vi "set MIC.maxpower.vi"() -> ()   [LabVIEW 2012]
uses:
  GFG/GFGnumericGet.vi
  GFG/GFG library.lvlib
panel:
  in  "OK Button":bool
  # "set half-wave plate to MAXIMUM power\nusing the control cube"
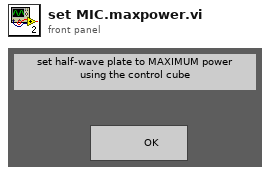
[diagram p1: front panel]
types:
  T1 = enum32{"Invalid", "Standard", "Closed", "Hidden", "Minimized", "Maximized"}
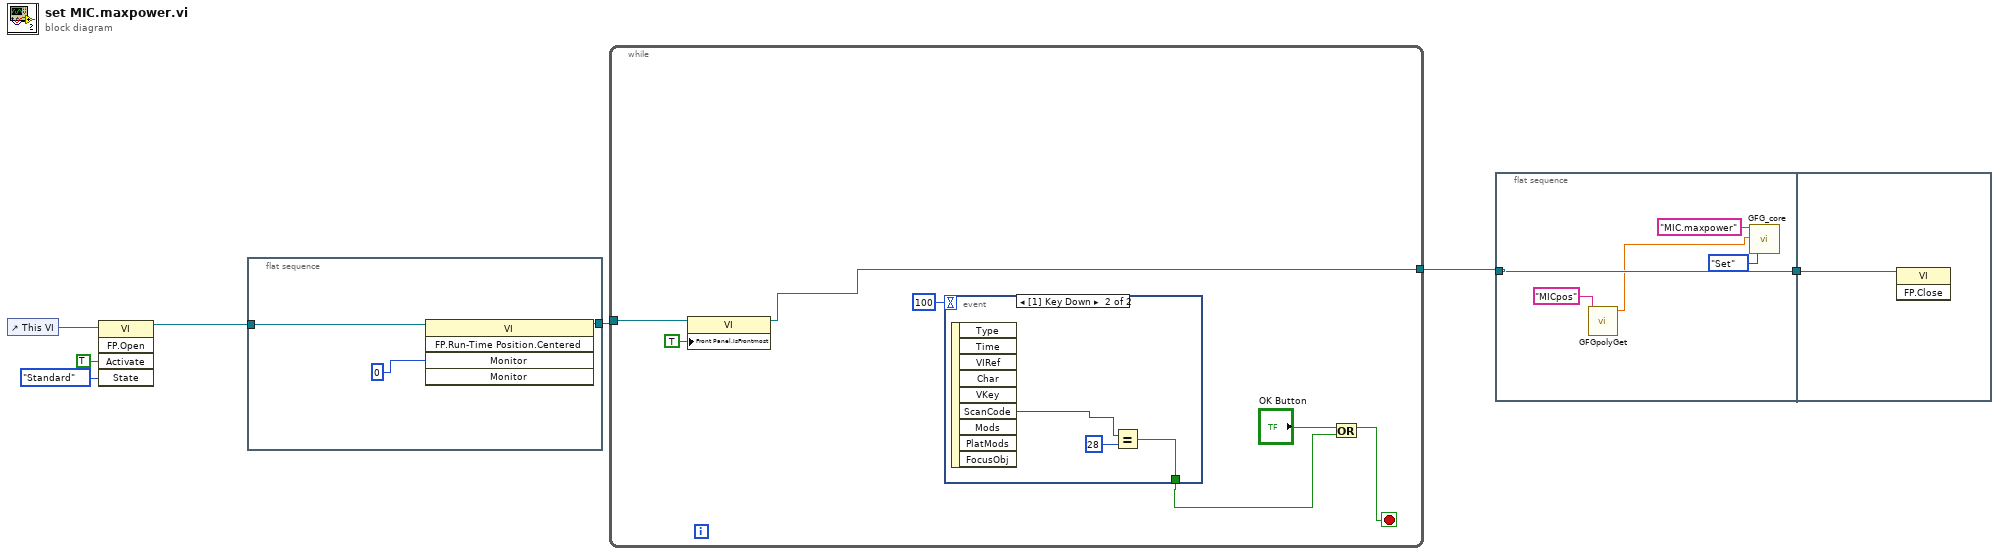
[diagram p0: block diagram]
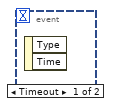
[diagram p2: hidden frame]
diagram:
  n1 = control-ref of="This VI"() -> (w5:refnum<vi>)
  n2 = invoke class="VI" method="FP.Open"(reference=w5, "Activate"=TRUE ("Activate?"), "State"=T1."Standard") -> (reference out=w2:refnum<vi>)  [unwired: 2 in, 4 out]
  n3 = flat-sequence {
    tunnel: [w9] -> w3
    tunnel: w2 -> [w8]
    frame #0 {
      n4 = invoke class="VI" method="FP.Run-Time Position.Centered"(reference=w8, "Monitor"=i16 0) -> (reference out=w9:refnum<vi>)  [unwired: 3 in, 4 out]
    }
  }
  n5 = while {
    tunnel: w3 -> [w14]
    tunnel: [w13] -> w4
    stop <- w12 stop-if-true
    n6 = property class="VI"(reference=w14, "Front Panel.IsFrontmost"=TRUE ("Front Panel Window:Is Frontmost")) -> (reference out=w13:refnum<vi>)  [unwired: 1 in, 1 out]
    n7 = event shown="[1] Key Down" {
      selector: _ -> [_ _]
      dyn-events: _ -> [_ _]
      timeout: 100 -> [_ _]
      tunnel: [_ w18] -> w11
      event Timeout {
        n8 = event-data() -> ()  [unwired: 1 in, 2 out]
      }
      event Key Down {
        n9 = event-data() -> ("ScanCode"=w20:i16)  [unwired: 1 in, 8 out]
        n10 = Equal?(x=w20, y=i16 28) -> (x = y?=w18:bool)
      }
    }
    n11 = Or(x="OK Button", y=w11) -> (x .or. y?=w12:bool)
  }
  n12 = flat-sequence {
    tunnel: w4 -> [w25]
    tunnel: [w25] -> w1
    tunnel: w1 -> [w26]
    frame #0 {
      n13 = call-poly "GFGpolyGet.vi"("Variable Name in"="MICpos") -> ("Numeric"=w21:dbl)  [unwired: 9 in, 1 out]
      n14 = call "GFG_core.vi"("Variable Name in"="MIC.maxpower", "Variant in"=w21, "Action"=enum16{"Init", "Set", "Get"}."Set") -> ()  [unwired: 10 in, 7 out]
    }
    frame #1 {
      n15 = invoke class="VI" method="FP.Close"(reference=w26) -> ()  [unwired: 2 in, 3 out]
    }
  }
